vi "Configure Motor (Output).vi"(0 "VISA resource name":refnum<visa-resource-name>, 2 "Scaling Factor (1.0000)":dbl=1.0 min=0.0001 max=99999.9999 format="%.4f", 11 "error in (no error)":errorcluster) -> (4 "VISA resource name out":refnum<visa-resource-name>, 15 "error out":errorcluster)   [LabVIEW 2021, in "Yokogawa WT1800 Series.lvlib"]
doc: "Configures the motor output features.\n\n<b>Note:</b>\nThis setting valid on models with the motor evaluation function (/MTR) option."
uses:
  <instrlib>/Yokogawa WT1800 Series/Yokogawa WT1800 Series.lvlib
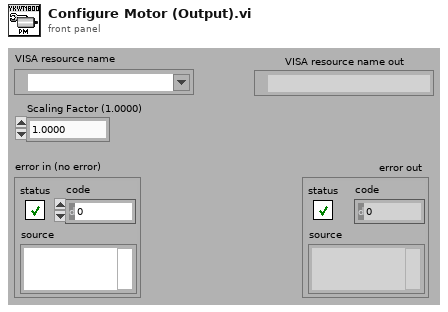
[diagram p1: front panel]
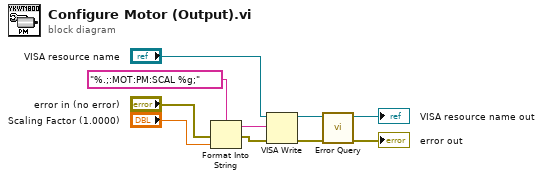
[diagram p0: block diagram]
diagram:
  n1 = Format Into String(format string="%.;:MOT:PM:SCAL %g;" ("形式文字列"), error in="error in (no error)", "Scaling Factor (1.0000)") -> (resulting string=w2:string, error out=w1:errorcluster)  [unwired: 1 in]
  n2 = VISA Write ("VISA書き込み")(VISA resource name="VISA resource name", write buffer=w2, error in (no error)=w1) -> (VISA resource name out=w10:refnum<visa-resource-name>, error out=w9:errorcluster)  [unwired: 1 out]
  n3 = call <instrlib>:"Error Query.vi"("error in (no error)"=w9, "VISA resource name"=w10) -> ("error out"=→"error out":errorcluster, "VISA resource name out"=→"VISA resource name out":refnum<visa-resource-name>)  [unwired: 6 in, 2 out]
